vi "SS_RESET_INIT.vi"(6 "Main Cluster IN":T1, 8 "Error In":errorcluster, 11 "Info In":string="\nWaiting for TimerScope Trigger\n- IN: SS TimerScope Trigger\n- OUT: SET SS ThermoRec Received Trigger\nPulse Number is 231123\nPulse Type is 4\n\nDuration (s) is  2.000000\nDelay (s)  is  1.000000\nScan Period (ms) is  15\nNumber of Samples is  134\n\nDelay Started\nDelay Complete\nExternal Measurement of Delay (s): 1.000000\nACQUIRING DATA") -> (0 "Error Out":errorcluster, 3 "Info Out":string="\nWaiting for TimerScope Trigger\n- IN: SS TimerScope Trigger\n- OUT: SET SS ThermoRec Received Trigger\nPulse Number is 231123\nPulse Type is 4\n\nDuration (s) is  2.000000\nDelay (s)  is  1.000000\nScan Period (ms) is  15\nNumber of Samples is  134\n\nDelay Started\nDelay Complete\nExternal Measurement of Delay (s): 1.000000\nACQUIRING DATA", 4 "Main Cluster OUT":T1)   [LabVIEW 2016]
uses:
  Control/Control_Main.ctl
  Control/Control_ModuleArray.ctl
panel:
  in  "Tab Control":enum32{"IN", "OUT", "SubVI Info"}(tab)
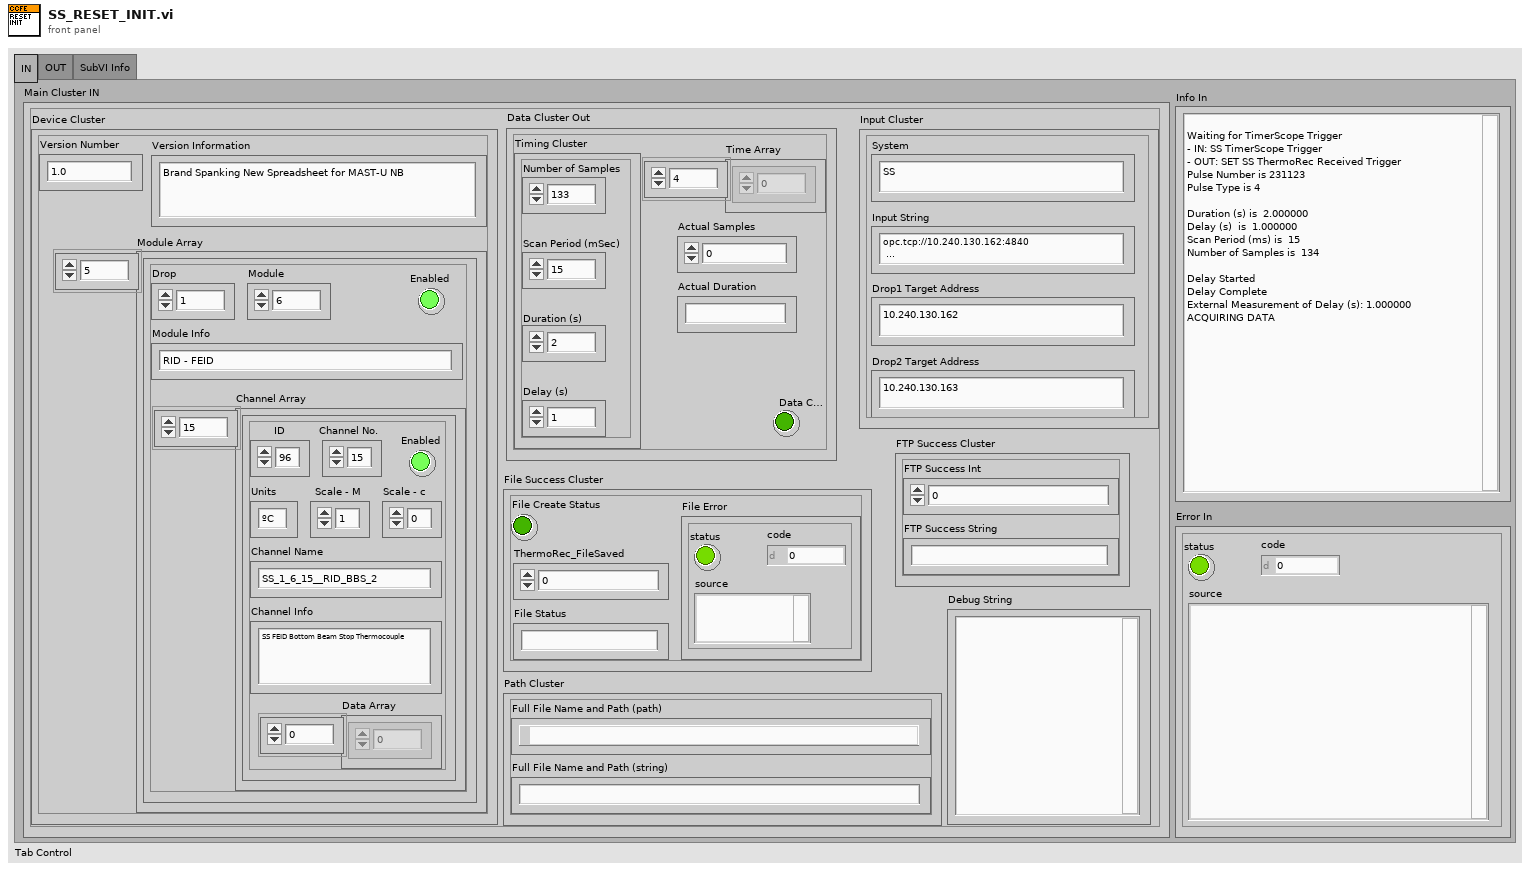
[diagram p1: front panel]
types:
  T1 = typedef "Control_Main.ctl" = cluster{"Device Cluster":cluster{"Module Array":T2, "Version Number":string, "Version Information":string}, "Input Cluster":cluster{"Input String":string, "Drop1 Target Address":string, "Drop2 Target Address":string, "System":string}, "Data Cluster Out":cluster{"Timing Cluster":cluster{"Number of Samples":i32, "Scan Period (mSec)":u32, "Duration (s)":dbl, "Delay (s)":dbl}, "Time Array":dbl[], "Actual Samples":i32, "Actual Duration":string, "Data Collection Error":bool}, "Path Cluster":cluster{"Full File Name and Path (path)":path, "Full File Name and Path (string)":string}, "File Success Cluster":cluster{"ThermoRec_FileSaved":i32, "File Create Status":bool, "File Error":errorcluster, "File Status":string}, "FTP Success Cluster":cluster{"FTP Success Int":i32, "FTP Success String":string}, "Debug String":string}
  T2 = typedef "Control_ModuleArray.ctl" = cluster{"Drop":i32, "Module":i32, "Module Info":string, "Enabled":bool, "Channel Array":cluster{"ID":i32, "Channel No.":i32, "Enabled":bool, "Channel Name":string, "Channel Info":string, "Units":string, "Scale - M":dbl, "Scale - c":dbl, "Data Array":dbl[]}[]}[]
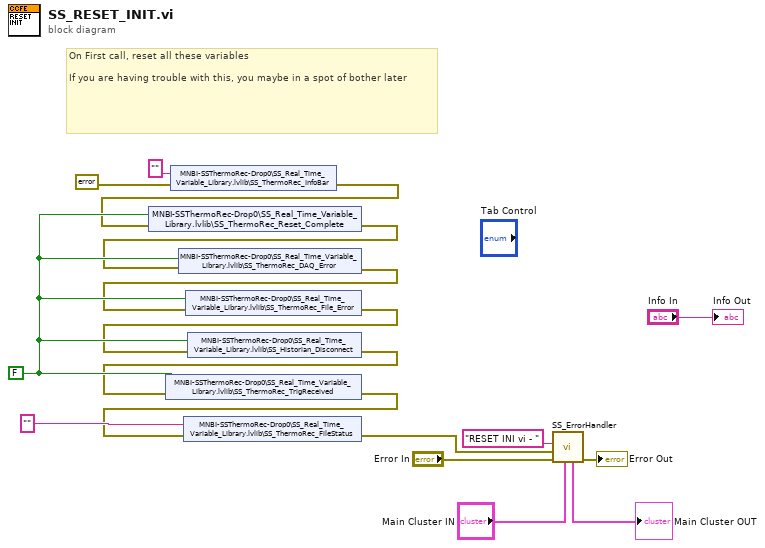
[diagram p0: block diagram]
diagram:
  w17 = FALSE ("SS_ThermoRec_TrigReceived")
  # "On First call, reset all these variables\n\nIf you are having trouble with this, you maybe in a spot of bother later"
  n1 = shared-variable "MNBI-SSThermoRec-Drop0\\SS_Real_Time_Variable_Library.lvlib\\SS_ThermoRec_InfoBar"("", error in=errorcluster {"status"=FALSE, "code"=0, "source"=""} ("error constant")) -> (error out=w1:errorcluster)
  n2 = shared-variable "MNBI-SSThermoRec-Drop0\\SS_Real_Time_Variable_Library.lvlib\\SS_ThermoRec_Reset_Complete"(w17, error in=w1) -> (error out=w16:errorcluster)
  n3 = shared-variable "MNBI-SSThermoRec-Drop0\\SS_Real_Time_Variable_Library.lvlib\\SS_ThermoRec_DAQ_Error"(w17, error in=w16) -> (error out=w15:errorcluster)
  n4 = shared-variable "MNBI-SSThermoRec-Drop0\\SS_Real_Time_Variable_Library.lvlib\\SS_ThermoRec_File_Error"(w17, error in=w15) -> (error out=w13:errorcluster)
  n5 = shared-variable "MNBI-SSThermoRec-Drop0\\SS_Real_Time_Variable_Library.lvlib\\SS_Historian_Disconnect"(w17, error in=w13) -> (error out=w14:errorcluster)
  n6 = shared-variable "MNBI-SSThermoRec-Drop0\\SS_Real_Time_Variable_Library.lvlib\\SS_ThermoRec_TrigReceived"(w17, error in=w14) -> (error out=w11:errorcluster)
  n7 = shared-variable "MNBI-SSThermoRec-Drop0\\SS_Real_Time_Variable_Library.lvlib\\SS_ThermoRec_FileStatus"("" ("SS_ThermoRec_FileStatus"), error in=w11) -> (error out=w7:errorcluster)
  n8 = call "SS_ErrorHandler.vi"("Main Cluster IN"="Main Cluster IN", "Error In"="Error In", "SubVI Error"=w7, "SubVI Name"="RESET INI vi - ") -> ("Error Out"=→"Error Out":errorcluster, "Main Cluster OUT"=→"Main Cluster OUT":T1)  [unwired: 5 in, 1 out]
  "Info Out" <- "Info In"
